vi "Joint Manipulator Inertia (Trajectory).vi"(8 "error in (no error)":errorcluster, 10 "joint position trajectory":dbl[][](array[numeric]), 11 "serial arm in":refnum<class "NI_Robotics_Serial Robot Arm.lvclass">) -> (0 "error out":errorcluster, 2 "inertia matrix trajectory":dbl[][][](array[numeric]), 3 "serial arm out":refnum<class "NI_Robotics_Serial Robot Arm.lvclass">)   [LabVIEW 2017, in "NI_Kinematics.lvlib"]
doc: "Calculates a matrix that represents the kinetic energy of the end effector of a robotic arm in joint space. Wire data to the <B>joint positions</B> input to determine the polymorphic instance to use or manually select the instance. \n\n<B>.m file:</B> inertia"
uses:
  <vilib>/robotics/Kinematics/NI_Kinematics.lvlib
  <vilib>/robotics/Kinematics/Robot/NI_Robotics_Serial Robot Arm.lvclass
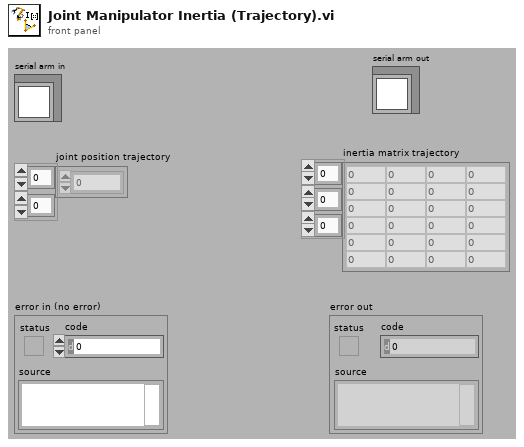
[diagram p1: front panel]
types:
  T1 = typedef "NI_Matrix.lvlib/RealMatrix.ctl" = dbl[][]
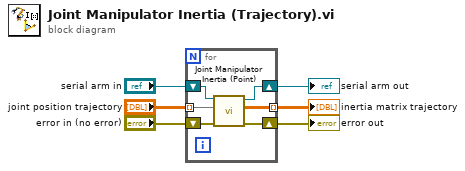
[diagram p0: block diagram]
diagram:
  n1 = for {
    tunnel: "joint position trajectory" -> [w12] mode=indexing
    tunnel: [w9] -> w3 mode=indexing
    shift-right: [w7] -> w1
    shift-left: "error in (no error)" -> [w8]
    shift-right: [w10] -> w4
    shift-left: "serial arm in" -> [w11]
    n2 = call <vilib>:"Joint Manipulator Inertia (Point).vi"("error in (no error)"=w8, "joint positions"=w12, "serial arm in"=w11) -> ("error out"=w7:errorcluster, "inertia matrix"=w9:T1, "serial arm out"=w10:refnum<class "NI_Robotics_Serial Robot Arm.lvclass">)  [unwired: 6 in]
  }
  "serial arm out" <- w4
  "inertia matrix trajectory" <- w3
  "error out" <- w1
